vi "Helmholtz2D_FEM_Delaunay_Area.vi"(6 "y3":dbl, 7 "x1":dbl, 8 "y2":dbl, 9 "y1":dbl, 10 "x3":dbl, 11 "x2":dbl) -> (3 "area":dbl)   [LabVIEW 2017, in "NI_PDE.lvlib"]
uses:
  <vilib>/gmath/NI_PDE.lvlib
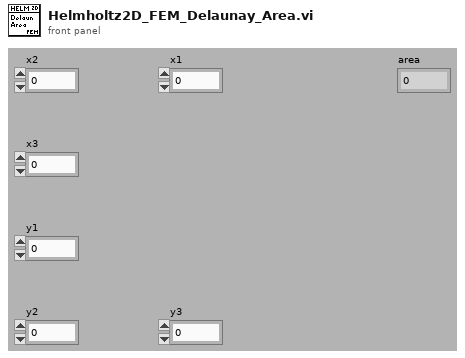
[diagram p1: front panel]
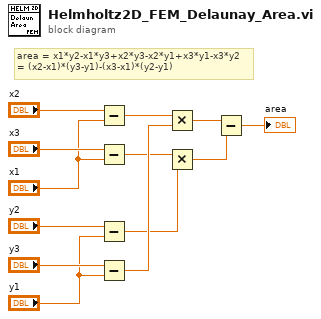
[diagram p0: block diagram]
diagram:
  # "area = x1*y2-x1*y3+x2*y3-x2*y1+x3*y1-x3*y2\n= (x2-x1)*(y3-y1)-(x3-x1)*(y2-y1)"
  n1 = Subtract(x="x2", y="x1") -> (x-y=w13:dbl)
  n2 = Subtract(x="x3", y="x1") -> (x-y=w10:dbl)
  n3 = Subtract(x="y2", y="y1") -> (x-y=w8:dbl)
  n4 = Subtract(x="y3", y="y1") -> (x-y=w12:dbl)
  n5 = Multiply(x=w13, y=w12) -> (x*y=w11:dbl)
  n6 = Multiply(x=w10, y=w8) -> (x*y=w9:dbl)
  n7 = Subtract(x=w11, y=w9) -> (x-y=→"area":dbl)
